vi "full adder.vi"() -> ()   [LabVIEW 2018]
panel:
  in  "FULL ADDER":string[][](table)=[["A", "B", "C", "SUM", "Cout"], ["0", "0", "0", "0", "0"], ["0", "0", "1", "1", "0"], ["0", "1", "0", "1", "0"], ["0", "1", "1", "0", "1"], ["1", "0", "0", "1", "0"], ["1", "0", "1", "0", "1"], ["1", "1", "0", "0", "1"], ["1", "1", "1", "1", "1"]]
  out "Cout":bool
  out "SUM":bool
  in  "B":bool
  in  "A":bool
  in  "Cin":bool
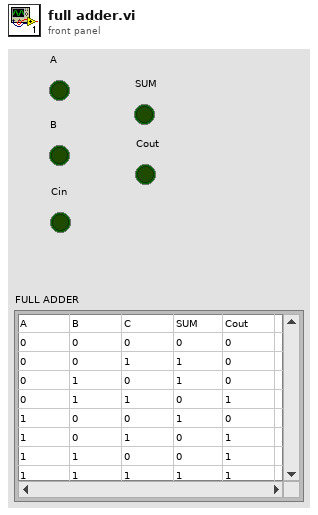
[diagram p1: front panel]
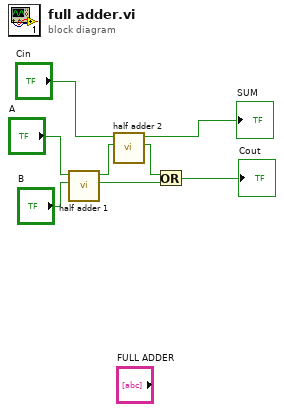
[diagram p0: block diagram]
diagram:
  n1 = call "half adder 1.vi"("B"="B", "A"="A") -> ("Boolean"=w2:bool, "Boolean 2"=w5:bool)  [unwired: 8 in]
  n2 = call "half adder 2.vi"("Boolean 3"=w5, "Cin"="Cin") -> ("Boolean"=w3:bool, "Boolean 2"=→"SUM":bool)  [unwired: 8 in]
  n3 = Or(x=w3, y=w2) -> (x .or. y?=→"Cout":bool)
